vi "Calc Bounds.vi"(11 "State":T4) -> (0 "Name Width":i16, 1 "Collapsed":i32, 2 "Header":i32, 3 "Text Bounds":T2, 4 "Name Center":i16, 5 "Bounds Without Terminals":T1, 7 "Full Bounds":T1)   [LabVIEW 2020, in "Parallel Diagram Block.xnode"]
uses:
  Parallel Diagram Block.xnode
  State.ctl
  Parallel Block/Type Descriptor.ctl
  Parallel Block/Direction.ctl
  Parallel Block/Value Type.ctl
  Parallel Block/Terminal Mode.ctl
  Parallel Block/Terminal Type.ctl
  Parallel Block/Type Mode.ctl
  Parallel Block/Value Mode.ctl
  <vilib>/picture/picture.llb/imagedata.ctl
  Parallel Block/Manager Node.ctl
  <vilib>/XNodeSupport/XNodeBounds.ctl
  <vilib>/XNodeSupport/XNodeInt.ctl
  <vilib>/XNodeSupport/NI_XNodeSupport.lvlib
  Parallel Block/Parallel Block.lvlib
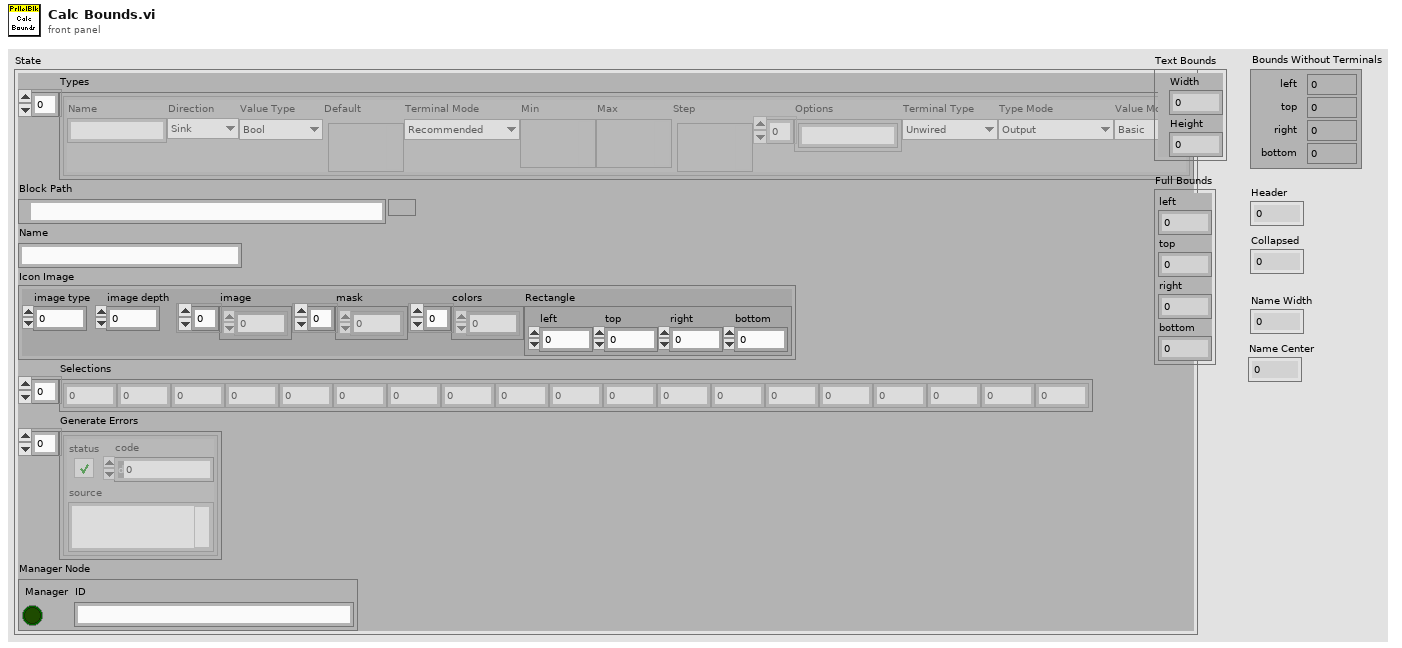
[diagram p1: front panel]
types:
  T1 = cluster{"left":i16, "top":i16, "right":i16, "bottom":i16}
  T2 = typedef "NI_XNodeSupport.lvlib/XNodeBounds.ctl" = cluster{"Width":T3, "Height":T3}
  T3 = typedef "NI_XNodeSupport.lvlib/XNodeInt.ctl" = i32
  T4 = typedef "Parallel Diagram Block.xnode/State.ctl" = cluster{"Types":T5[], "Block Path":path, "Name":string, "Icon Image":T12, "Selections":i32[], "Generate Errors":errorcluster[], "Manager Node":T13}
  T5 = typedef "Parallel Block.lvlib/Type Descriptor.ctl" = cluster{"Name":string, "Direction":T6, "Value Type":T7, "Default":variant, "Terminal Mode":T8, "Min":variant, "Max":variant, "Step":variant, "Options":string[], "Terminal Type":T9, "Type Mode":T10, "Value Mode":T11}
  T6 = typedef "Parallel Block.lvlib/Direction.ctl" = enum16{"Sink", "Source"}
  T7 = typedef "Parallel Block.lvlib/Value Type.ctl" = enum16{"Unknown", "Bool", "U8", "U16", "U32", "U64", "I8", "I16", "I32", "I64", "SGL", "DBL", "CSG", "CDB", "CDBWfm", "String", "DBLWfm"}
  T8 = typedef "Parallel Block.lvlib/Terminal Mode.ctl" = enum16{"Recommended", "Required", "None"}
  T9 = typedef "Parallel Block.lvlib/Terminal Type.ctl" = enum16{"Unwired", "BadType", "Connection", "Value", "Control Ref", "BadRefType"}
  T10 = typedef "Parallel Block.lvlib/Type Mode.ctl" = enum16{"Output", "Single - Strict", "Single - Coerced", "Stream"}
  T11 = typedef "Parallel Block.lvlib/Value Mode.ctl" = enum16{"Basic", "Range", "Select"}
  T12 = typedef "imagedata.ctl" = cluster{"image type":i32, "image depth":i32, "image":u8[], "mask":u8[], "colors":u32[], "Rectangle":cluster{"left":i16, "top":i16, "right":i16, "bottom":i16}}
  T13 = typedef "Parallel Block.lvlib/Manager Node.ctl" = cluster{"Manager":bool, "ID":string}
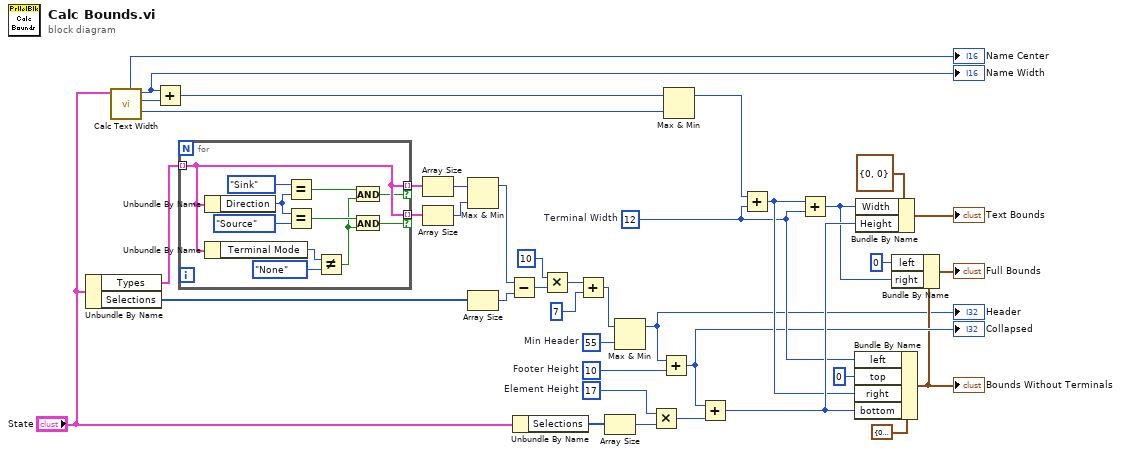
[diagram p0: block diagram]
diagram:
  w16 = 55  # Min Header
  w29 = 12  # Terminal Width
  w28 = 10  # Footer Height
  w39 = 17  # Element Height
  n1 = Unbundle By Name("State") -> ("Types"=w13:T5[], "Selections"=w19:i32[])
  n2 = call "Calc Text Width.vi"("State"="State") -> ("Value Width"=w4:i16, "Name Width"=w6:i16, "Name Center"=→"Name Center":i16, "Min Width"=w1:i16)  [unwired: 7 in]
  "Name Width" <- w6
  n3 = Add(x=w6, y=w4) -> (x+y=w5:i16)
  n4 = for {
    tunnel: w13 -> [w45] mode=indexing
    tunnel: [w45] -> w12 mode=indexing if=w41
    tunnel: [w45] -> w11 mode=indexing if=w42
    n5 = Unbundle By Name(w45) -> ("Direction"=w48:T6)
    n6 = Unbundle By Name(w45) -> ("Terminal Mode"=w44:T8)
    n7 = Equal?(x=Direction."Sink", y=w48) -> (x = y?=w47:bool)
    n8 = Equal?(x=w48, y=Direction."Source" ("x")) -> (x = y?=w46:bool)
    n9 = Not Equal?(x=w44, y=Terminal_Mode."None") -> (x != y?=w40:bool)
    n10 = And(x=w47, y=w40) -> (x .and. y?=w41:bool)
    n11 = And(x=w46, y=w40) -> (x .and. y?=w42:bool)
  }
  n12 = Array Size(array=w12) -> (size(s)=w10:i32)
  n13 = Array Size(array=w11) -> (size(s)=w9:i32)
  n14 = Max & Min(x=w10, y=w9) -> (max(x,y)=w8:i32)  [unwired: 1 out]
  n15 = Array Size(array=w19) -> (size(s)=w18:i32)
  n16 = Subtract(x=w8, y=w18) -> (x-y=w17:i32)
  n17 = Unbundle By Name("State") -> ("Selections"=w37:i32[])
  n18 = Multiply(x=10 ("y"), y=w17) -> (x*y=w22:i32)
  n19 = Add(x=w22, y=7) -> (x+y=w14:i32)
  n20 = Array Size(array=w37) -> (size(s)=w36:i32)
  n21 = Max & Min(x=w14, y=w16) -> (max(x,y)=w15:i32)  [unwired: 1 out]
  "Header" <- w15
  n22 = Multiply(x=w39, y=w36) -> (x*y=w38:i32)
  n23 = Add(x=w15, y=w28) -> (x+y=w27:i32)
  "Collapsed" <- w27
  n24 = Max & Min(x=w5, y=w1) -> (max(x,y)=w2:i16)  [unwired: 1 out]
  n25 = Add(x=w27, y=w38) -> (x+y=w32:i32)
  n26 = Add(x=w2, y=w29) -> (x+y=w30:i32)
  n27 = Add(x=w30, y=w29) -> (x+y=w25:i32)
  n28 = Bundle By Name(cluster=T1 {"left"=0, "top"=0, "right"=0, "bottom"=0} ("Border Without Terminals"), "left"=w29, "top"=i16 0, "right"=w30, "bottom"=w32) -> (w24:T1)
  "Bounds Without Terminals" <- w24
  n29 = Bundle By Name(cluster=T2 {"Width"=0, "Height"=0} ("Bounds"), "Width"=w25, "Height"=w32) -> (→"Text Bounds":T2)
  n30 = Bundle By Name(cluster=w24, "left"=i16 0, "right"=w25) -> (→"Full Bounds":T1)
